vi "Global Variables.vi"() -> ()   [LabVIEW 2011]
panel:
  out "Full String_global":string
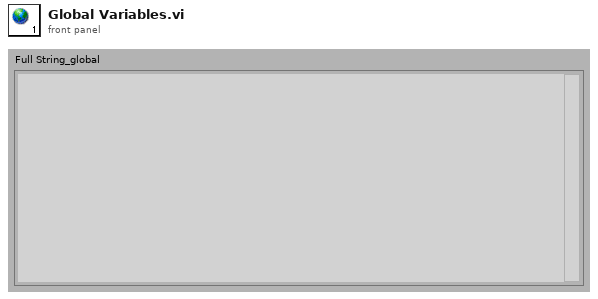
[diagram p1: front panel]
diagram:
